vi "Wait.vi"(8 "error in (no error)":errorcluster, 11 "BiStableShutter in":refnum<class "BiStableShutter.lvclass">) -> (0 "error out":errorcluster, 2 "State":T1, 3 "BiStableShutter out":refnum<class "BiStableShutter.lvclass">)   [LabVIEW 2016, in "BiStableShutter.lvclass"]
uses:
  BiStableShutter.lvclass
  Controls/Shutter States.ctl
  BiStableShutter.lvclass/BiStableShutter.ctl
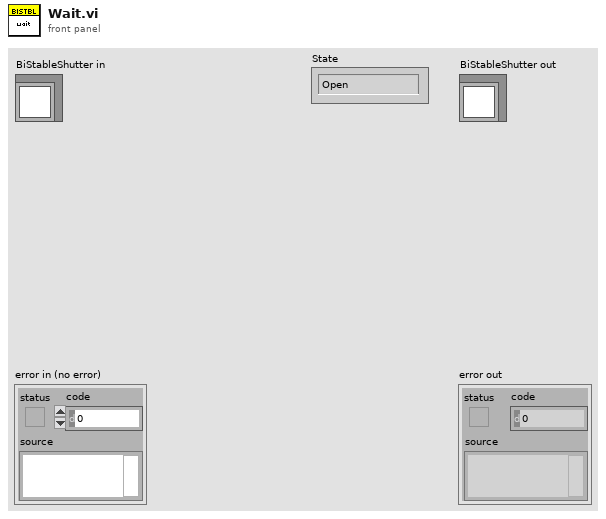
[diagram p1: front panel]
types:
  T1 = typedef "Shutter States.ctl" = enum16{"Open", "Close", "Wait", "Off", "Arm", "Idle"}
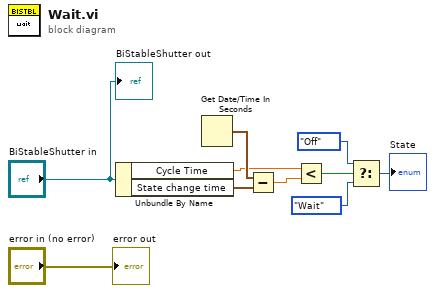
[diagram p0: block diagram]
diagram:
  n1 = Unbundle By Name("BiStableShutter in") -> ("Cycle Time"=w5:dbl, "State change time"=w1:timestamp)
  n2 = Get Date/Time In Seconds() -> (seconds since 1Jan1904=w8:timestamp)
  n3 = Subtract(x=w8, y=w1) -> (x-y=w4:dbl)
  n4 = Less?(x=w5, y=w4) -> (x < y?=w3:bool)
  n5 = Select(t=Shutter_States."Off" ("State"), s=w3, f=Shutter_States."Wait") -> (s? t:f=→"State":T1)
  "error out" <- "error in (no error)"
  "BiStableShutter out" <- "BiStableShutter in"
